vi "Gamepad NanoDrive Control.vi"() -> ()   [LabVIEW 2012]
uses:
  <vilib>/Utility/miscctls.llb/LVPointTypeDef.ctl
  <vilib>/Utility/file.llb/Read From Spreadsheet File (I64).vi
  <vilib>/Utility/inputDevices.llb/joystickAcquire.vi
  <vilib>/Utility/inputDevices.llb/closeJoystick.vi
  Madlib.dll
panel:
  out "Y axis":dbl
  out "X axis":dbl
  out "yRead":dbl=5.0 step=0.1 format="%.3f"
  out "xRead":dbl=5.0 step=0.1 format="%.3f"
  in  "left":bool
  in  "down":bool
  in  "right":bool
  in  "up":bool
  in  "closed?":bool
  in  "Slide":cluster{u32, u32}(slide)={0, 5} scale=0.0..7.0
  in  "configure":bool
  out "button selection refs":T1
  in  "yf":u16(ring)=4 items=["1 X"=1, "2 A"=2, "3 B"=3, "4 Y"=4, "5 LB"=5, "6 RB"=6, "7 LT"=7, "8 RT"=8, "9 Back"=9]
  in  "xf":u16(ring)=3 items=["1 X"=1, "2 A"=2, "3 B"=3, "4 Y"=4, "5 LB"=5, "6 RB"=6, "7 LT"=7, "8 RT"=8, "9 Back"=9]
  in  "yf xr 2":u16(ring)=5 items=["1 X"=1, "2 A"=2, "3 B"=3, "4 Y"=4, "5 LB"=5, "6 RB"=6, "7 LT"=7, "8 RT"=8, "9 Back"=9]
  in  "halt 3":u16(ring)=9 items=["1 X"=1, "2 A"=2, "3 B"=3, "4 Y"=4, "5 LB"=5, "6 RB"=6, "7 LT"=7, "8 RT"=8, "9 Back"=9]
  in  "yf xf 2":u16(ring)=6 items=["1 X"=1, "2 A"=2, "3 B"=3, "4 Y"=4, "5 LB"=5, "6 RB"=6, "7 LT"=7, "8 RT"=8, "9 Back"=9]
  in  "yr xr 2":u16(ring)=7 items=["1 X"=1, "2 A"=2, "3 B"=3, "4 Y"=4, "5 LB"=5, "6 RB"=6, "7 LT"=7, "8 RT"=8, "9 Back"=9]
  in  "yr":u16(ring)=2 items=["1 X"=1, "2 A"=2, "3 B"=3, "4 Y"=4, "5 LB"=5, "6 RB"=6, "7 LT"=7, "8 RT"=8, "9 Back"=9]
  in  "yr xf 2":u16(ring)=8 items=["1 X"=1, "2 A"=2, "3 B"=3, "4 Y"=4, "5 LB"=5, "6 RB"=6, "7 LT"=7, "8 RT"=8, "9 Back"=9]
  in  "xr":u16(ring)=1 items=["1 X"=1, "2 A"=2, "3 B"=3, "4 Y"=4, "5 LB"=5, "6 RB"=6, "7 LT"=7, "8 RT"=8, "9 Back"=9]
  in  "down-left":bool
  in  "down-right":bool
  in  "up-left":bool
  in  "up-right":bool
  in  "yStep":dbl=1.0 min=0.01905 max=4.0 format="%.3f"
  in  "xStep":dbl=1.0 min=0.01905 max=4.0 format="%.3f"
  in  "Invert":bool=TRUE
  in  "Invert":bool
  # "Single Step Controls"
  # "Position"
  # "Step distance"
  # "Current position"
  # "X axis"
  # "X axis"
  # "um"
  # "um"
  # "Y axis"
  # "Y axis"
  # "um"
  # "um"
  # "Step"
  # "Commanded position"
  # "um"
  # "um"
  # "Configuration"
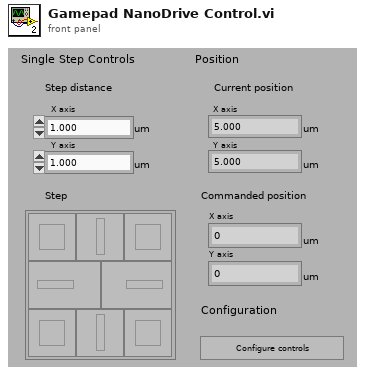
[diagram p1: front panel]
types:
  T1 = cluster{"xr":refnum<vi>, "yr":refnum<vi>, "xf":refnum<vi>, "yf":refnum<vi>, "yf xr 2":refnum<vi>, "yf xf 2":refnum<vi>, "yr xr 2":refnum<vi>, "yr xf 2":refnum<vi>, "halt 2":refnum<vi>}
  T2 = enum16{"open", "replace", "create", "open or create", "replace or create", "replace or create with confirmation"}
  T3 = typedef "LVPointTypeDef.ctl" = cluster{"Horizontal":i16, "Vertical":i16}
  T4 = cluster{"Controls":cluster{"Commands":cluster{"unused":bool}, "Values":cluster{"up":u16, "right":u16}}, "ControlRefs":cluster{"Commands":cluster{"unused":refnum<vi>}, "Values":cluster{"up":refnum<vi>, "right":refnum<vi>}}, "Variables":cluster{"Commands":cluster{"up_changed":bool, "right_changed":bool}, "Values":cluster{"unused":i32}}}
  T5 = cluster{"Controls":cluster{"Commands":cluster{"right":bool, "left":bool, "up":bool, "down":bool, "down-left":bool, "up-left":bool, "up-right":bool, "down-right":bool}, "Values":cluster{"xStep":dbl, "yStep":dbl, "xRead":dbl, "yRead":dbl}}, "ControlRefs":cluster{"Commands":cluster{"right":refnum<vi>, "left":refnum<vi>, "up":refnum<vi>, "down":refnum<vi>, "down-left":refnum<vi>, "up-left":refnum<vi>, "up-right":refnum<vi>, "down-right":refnum<vi>}, "Values":cluster{"X step":refnum<vi>, "Y step":refnum<vi>, "xRead":refnum<vi>, "yRead":refnum<vi>}}, "Variables":cluster{"Commands":cluster{"unused":bool}, "Values":cluster{"xCommand":dbl, "yCommand":dbl, "xCalibration":dbl, "yCalibration":dbl}}}
  T6 = cluster{"xr":refnum<vi>, "yr":refnum<vi>, "xf":refnum<vi>, "yf":refnum<vi>, "yf xr 2":refnum<vi>, "yf xf 2":refnum<vi>, "yr xr 2":refnum<vi>, "yr xf 2":refnum<vi>, "halt 3":refnum<vi>}
  T7 = cluster{"X axis":i32, "Y axis":i32, "Z axis":i32, "X axis rotation":i32, "Y axis rotation":i32, "Z axis rotation":i32, "U axis":i32, "V axis":i32}
  T8 = cluster{"button 1":bool, "button 2":bool, "button 3":bool, "button 4":bool, "button 5":bool, "button 6":bool, "button 7":bool, "button 8":bool, "button 9":bool, "button 10":bool, "button 11":bool, "button 12":bool, "button 13":bool, "button 14":bool, "button 15":bool, "button 16":bool, "button 17":bool, "button 18":bool, "button 19":bool, "button 20":bool, "button 21":bool, "button 22":bool, "button 23":bool, "button 24":bool, "button 25":bool, "button 26":bool, "button 27":bool, "button 28":bool, "button 29":bool, "button 30":bool, "button 31":bool, "button 32":bool}
  T9 = cluster{"left":bool, "down":bool, "right":bool, "up":bool, "up-left":bool, "up-right":bool, "down-left":bool, "down-right":bool, "halt":bool, "button 10":bool}
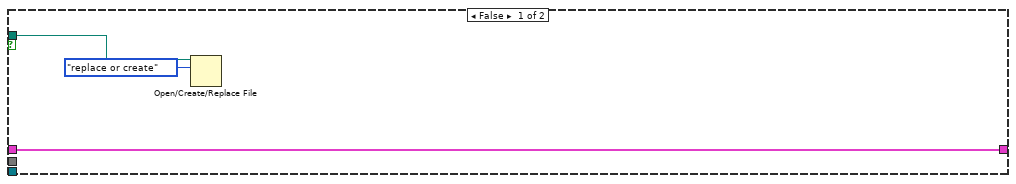
[diagram p2: hidden frame]
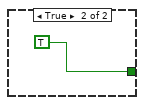
[diagram p4: hidden frame]
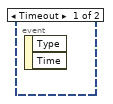
[diagram p8: hidden frame]
diagram:
  n1 = flat-sequence {
    tunnel: [w44] -> w25
    tunnel: [w43] -> w24
    tunnel: [w42] -> w23
    tunnel: [w61] -> w17
    tunnel: [w60] -> w16
    tunnel: [w59] -> w15
    tunnel: w25 -> [w61]
    tunnel: w24 -> [w56]
    tunnel: w23 -> [w59]
    tunnel: w17 -> [w64]
    tunnel: [w63] -> w27
    tunnel: w16 -> [w74]
    tunnel: [w74] -> w26
    tunnel: w15 -> [w62]
    tunnel: [w62] -> w22
    tunnel: w27 -> [w80]
    tunnel: [w80] -> w29
    tunnel: w26 -> [w86]
    tunnel: [w86] -> w28
    tunnel: w22 -> [w77]
    tunnel: [w76] -> w19
    tunnel: [w135] -> w35
    tunnel: [w136] -> w31
    tunnel: w28 -> [w136]
    tunnel: w29 -> [w135]
    tunnel: [w128] -> w20
    tunnel: w19 -> [w128]
    tunnel: [w141] -> w38
    tunnel: [w140] -> w37
    tunnel: w35 -> [w139]
    tunnel: [w139] -> w34
    tunnel: [w138] -> w32
    tunnel: w31 -> [w138]
    tunnel: [w137] -> w21
    tunnel: w20 -> [w137]
    tunnel: [w167] -> w12
    tunnel: [w168] -> w10
    tunnel: [w164] -> w8
    tunnel: w38 -> [w168]
    tunnel: w37 -> [w167]
    tunnel: w34 -> [w163]
    tunnel: [w163] -> w6
    tunnel: w32 -> [w162]
    tunnel: [w162] -> w4
    tunnel: w21 -> [w161]
    tunnel: [w161] -> w2
    tunnel: w12 -> [w190]
    tunnel: [w190] -> w11
    tunnel: w10 -> [w189]
    tunnel: [w189] -> w9
    tunnel: w8 -> [w185]
    tunnel: [w185] -> w7
    tunnel: w6 -> [w184]
    tunnel: [w184] -> w5
    tunnel: w4 -> [w183]
    tunnel: [w180] -> w3
    tunnel: w2 -> [w188]
    tunnel: [w188] -> w1
    tunnel: w11 -> [w197]
    tunnel: [w197] -> w41
    tunnel: w9 -> [w198]
    tunnel: [w198] -> w40
    tunnel: w7 -> [w196]
    tunnel: [w196] -> w39
    tunnel: [u32 0 ("current button state")] -> w36
    tunnel: [w193] -> w33
    tunnel: w5 -> [w193]
    tunnel: [w192] -> w30
    tunnel: w3 -> [w192]
    tunnel: [w191] -> w18
    tunnel: w1 -> [w191]
    tunnel: w39 -> [w205]
    tunnel: w40 -> [w207]
    tunnel: w41 -> [w206]
    tunnel: w36 -> [w204]
    tunnel: w33 -> [w203]
    tunnel: w30 -> [w202]
    tunnel: w18 -> [w201]
    tunnel: [w200] -> w14
    tunnel: [w199] -> w13
    tunnel: w14 -> [w489]
    tunnel: w13 -> [w488]
    frame #0 {
      w42 = T4 {"Controls"={"Commands"={"unused"=FALSE}, "Values"={"up"=2, "right"=0}}, "ControlRefs"={"Commands"={"unused"=refnum}, "Values"={"up"=refnum, "right"=refnum}}, "Variables"={"Commands"={"up_changed"=FALSE, "right_changed"=FALSE}, "Values"={"unused"=0}}}  # Configuration
      w43 = T5 {"Controls"={"Commands"={"right"=FALSE, "left"=FALSE, "up"=FALSE, "down"=FALSE, "down-left"=FALSE, "up-left"=FALSE, "up-right"=FALSE, "down-right"=FALSE}, "Values"={"xStep"=1.0, "yStep"=1.0, "xRead"=1.0, "yRead"=1.0}}, "ControlRefs"={"Commands"={"right"=refnum, "left"=refnum, "up"=refnum, "down"=refnum, "down-left"=refnum, "up-left"=refnum, "up-right"=refnum, "down-right"=refnum}, "Values"={"X step"=refnum, "Y step"=refnum, "xRead"=refnum, "yRead"=refnum}}, "Variables"={"Commands"={"unused"=FALSE}, "Values"={"xCommand"=0.0, "yCommand"=0.0, "xCalibration"=0.0, "yCalibration"=0.0}}}  # Motion
      w44 = T6 {"xr"=refnum, "yr"=refnum, "xf"=refnum, "yf"=refnum, "yf xr 2"=refnum, "yf xf 2"=refnum, "yr xr 2"=refnum, "yr xf 2"=refnum, "halt 3"=refnum}  # output cluster
    }
    frame #1 {
      n2 = control-ref of="right"() -> (w54:refnum<vi>)
      n3 = control-ref of="left"() -> (w53:refnum<vi>)
      n4 = control-ref of="up"() -> (w52:refnum<vi>)
      n5 = control-ref of="down"() -> (w51:refnum<vi>)
      n6 = control-ref of="down-left"() -> (w50:refnum<vi>)
      n7 = control-ref of="up-left"() -> (w49:refnum<vi>)
      n8 = control-ref of="up-right"() -> (w48:refnum<vi>)
      n9 = control-ref of="down-right"() -> (w47:refnum<vi>)
      n10 = control-ref of="xStep"() -> (w57:refnum<vi>)
      n11 = control-ref of="yStep"() -> (w58:refnum<vi>)
      n12 = control-ref of="xRead"() -> (w46:refnum<vi>)
      n13 = control-ref of="yRead"() -> (w45:refnum<vi>)
      n14 = Bundle By Name(cluster=w56, "ControlRefs.Values.X step"=w57, "ControlRefs.Values.Y step"=w58, "ControlRefs.Values.xRead"=w46, "ControlRefs.Values.yRead"=w45) -> (w55:T5)
      n15 = Bundle By Name(cluster=w55, "ControlRefs.Commands.right"=w54, "ControlRefs.Commands.left"=w53, "ControlRefs.Commands.up"=w52, "ControlRefs.Commands.down"=w51, "ControlRefs.Commands.down-left"=w50, "ControlRefs.Commands.up-left"=w49, "ControlRefs.Commands.up-right"=w48, "ControlRefs.Commands.down-right"=w47) -> (w60:T5)
    }
    frame #2 {
      n16 = control-ref of="xr"() -> (w73:refnum<vi>)
      n17 = control-ref of="yr"() -> (w72:refnum<vi>)
      n18 = control-ref of="xf"() -> (w71:refnum<vi>)
      n19 = control-ref of="yf"() -> (w70:refnum<vi>)
      n20 = control-ref of="yf xr 2"() -> (w69:refnum<vi>)
      n21 = control-ref of="yf xf 2"() -> (w68:refnum<vi>)
      n22 = control-ref of="yr xr 2"() -> (w67:refnum<vi>)
      n23 = control-ref of="yr xf 2"() -> (w66:refnum<vi>)
      n24 = control-ref of="halt 3"() -> (w65:refnum<vi>)
      n25 = Bundle(cluster=w64, "xr"=w73, "yr"=w72, "xf"=w71, "yf"=w70, "yf xr 2"=w69, "yf xf 2"=w68, "yr xr 2"=w67, "yr xf 2"=w66, "halt 3"=w65) -> (w63:T6)
    }
    frame #3 {
      n26 = control-ref of="This Application"() -> (w85:refnum<vi>)
      n27 = property class="App"(reference=w85) -> ("App.Dir"=w79:path)  [unwired: 1 in, 2 out]
      n28 = control-ref of="Slide"() -> (w82:refnum<vi>)
      n29 = Build Path(base path=w79, name or relative path="config.txt") -> (appended path=w83:path)
      n30 = Cluster To Array(cluster=w80) -> (array=w81:refnum<vi>[])
      n31 = call <vilib>:"Check if File or Folder Exists.vi"("path"=w83) -> ("file or folder exists?"=w75:bool, "dup path"=w78:path)  [unwired: 1 in, 8 out]
      n32 = case shown="True" w75 {
        tunnel: w82 -> [_ w103]
        tunnel: w81 -> [_ w102]
        tunnel: w78 -> [w89 w101]
        tunnel: w77 -> [w87 w91]
        tunnel: [w87 w90] -> w76
        frame False {
          n33 = Open/Create/Replace File(file path (use dialog)=w89, operation (0:open)=T2."replace or create") -> ()  [unwired: 1 in, 6 out]
        }
        frame True {
          n34 = Read from Text File(file (use dialog)=w101) -> (text=w100:string)  [unwired: 1 in, 5 out]
          n35 = String To Path(string=w100) -> (path=w99:path)
          n36 = call <vilib>:"Check if File or Folder Exists.vi"("path"=w99) -> ("file or folder exists?"=w97:bool, "dup path"=w93:path)  [unwired: 1 in, 8 out]
          n37 = Not A Number/Path/Refnum?(number/path/refnum=w93) -> (NaN/Path/Refnum?=w96:bool)
          n38 = Empty String/Path?(string/path=w93) -> (empty?=w94:bool)
          n39 = Not(x=w96) -> (.not. x?=w95:bool)
          n40 = Not(x=w94) -> (.not. x?=w92:bool)
          n41 = Compound Arithmetic op=AND(w95, w97, w92) -> (w98:bool)
          n42 = case shown="True" w98 {
            tunnel: w102 -> [_ w122]
            tunnel: w103 -> [_ w123]
            tunnel: w93 -> [_ w121]
            tunnel: w91 -> [w104 w120]
            tunnel: [w104 w119] -> w90
            frame False {
            }
            frame True {
              n43 = call-poly <vilib>:"Read From Spreadsheet File.vi"("transpose (no:F)"=TRUE ("transpose? (no:F)"), "file path (dialog if empty)"=w121) -> ("first row"=w124:i64[])  [unwired: 2 in, 7 out]
              n44 = Array Size(array=w122) -> (size(s)=w118:i32)
              n45 = Split 1D Array(array=w124, index=w118) -> (first subarray=w115:i64[], second subarray=w117:i64[])
              n46 = Index Array(array=w117) -> (element #1=w107:i64, element #2=w108:i64, element #3=w114:i64, element #4=w111:i64, element #5=w106:i64, element #6=w105:i64)  [unwired: 6 in]
              n47 = Bundle(w108, w107) -> (w116:cluster{i64, i64})  [unwired: 1 out]
              n48 = property class="Slide (strict)"(reference=w123, "Value"=w116) -> ()  [unwired: 1 in, 2 out]
              n49 = Bundle By Name(cluster=w120, "Controls.Values.up"=w106, "Controls.Values.right"=w105) -> (w119:T4)
              n50 = control-ref of="Invert"() -> (w110:refnum<vi>)
              n51 = control-ref of="Invert"() -> (w109:refnum<vi>)
              n52 = Greater Than 0?(x=w114) -> (x > 0?=w113:bool)
              n53 = Greater Than 0?(x=w111) -> (x > 0?=w112:bool)
              n54 = property class="Bool (strict)"(reference=w110, "Value"=w113) -> ()  [unwired: 1 in, 2 out]
              n55 = property class="Bool (strict)"(reference=w109, "Value"=w112) -> ()  [unwired: 1 in, 2 out]
              n56 = for {
                tunnel: w122 -> [w127] mode=indexing
                tunnel: w115 -> [w126] mode=indexing
                n57 = property class="Ring (strict)"(reference=w127, "Value"=w126) -> ()  [unwired: 1 in, 2 out]
              }
            }
          }
        }
      }
    }
    frame #4 {
      w131 = TRUE ("Front Panel Window:Closeable")
      w132 = FALSE ("Front Panel Window:Title Bar Visible")
      n58 = control-ref of="Pane"() -> (w129:refnum<vi>)
      n59 = control-ref of="This VI"() -> (w134:refnum<vi>)
      n60 = property class="VI"(reference=w134, "Front Panel.Title"="Gamepad NanoDrive Control" ("Front Panel Window:Title"), "Front Panel.TitleBarVis"=w131, "TB.Visible"=w132, "Front Panel.ShowMenuBar"=w132, "Front Panel.Closeable"=w131) -> ()  [unwired: 1 in, 2 out]
      n61 = property class="Pane"(reference=w129, "Origin"=T3 {"Horizontal"=0, "Vertical"=0}) -> ()  [unwired: 1 in, 2 out]
    }
    frame #5 {
      n62 = while {
        tunnel: [w147] -> w140
        tunnel: [w142] -> w141
        stop <- w146 stop-if-true
        n63 = flat-sequence {
          tunnel: [w150] -> w149
          tunnel: [w151] -> w148
          tunnel: [w150] -> w145
          tunnel: w149 -> [w155]
          tunnel: [w154] -> w147
          tunnel: w148 -> [w154]
          tunnel: [w153] -> w142
          tunnel: w145 -> [w153]
          tunnel: [w152] -> w144
          frame #0 {
            n64 = call "init joystick.vi"() -> ("device ID"=w151:refnum<k1>, "Joystick found"=w150:bool)  [unwired: 2 out]
          }
          frame #1 {
            n65 = case shown="False" w155 {
              tunnel: [w156 TRUE ("T button?")] -> w152
              frame False {
                n66 = Two Button Dialog(message="Press start (button 10)\n on your Gamepad \n(while pressing 'Ok')\nfor it to be initialized. ", 1:"Cancel Program" ("F button name (\"Cancel\")"), 2:"Ok" ("T button name (\"OK\")")) -> (T button?=w156:bool)
              }
              frame True {
              }
            }
          }
        }
        n67 = Not(x=w144) -> (.not. x?=w143:bool)
        n68 = Or(x=w143, y=w142) -> (x .or. y?=w146:bool)
      }
    }
    frame #6 {
      n69 = dll-call lib="C:/Users/Labview/Desktop/SRR/Madlib_x64/Labview Examples/Madlib.dll" fn="MCL_InitHandleOrGetExisting"() -> ("return type"=w165:i32)  [unwired: 3 in, 2 out]
      n70 = Less Or Equal To 0?(x=w165) -> (x <= 0?=w166:bool)
      n71 = case shown="True" w166 {
        tunnel: w165 -> [w169 w171]
        tunnel: [w169 w170] -> w164
        frame False {
        }
        frame True {
          n72 = while {
            tunnel: w171 -> [w176]
            tunnel: [w174] -> w170
            stop <- w173 continue-if-true
            n73 = Two Button Dialog(message="Failed to load NanoDrive!\nReInit?") -> (T button?=w172:bool)  [unwired: 2 out]
            n74 = case shown="True" w172 {
              tunnel: w176 -> [w178 _]
              tunnel: [w178 w179] -> w174
              frame False {
              }
              frame True {
                n75 = dll-call lib="C:/Users/Labview/Desktop/SRR/Madlib_x64/Labview Examples/Madlib.dll" fn="MCL_InitHandleOrGetExisting"() -> ("return type"=w179:i32)  [unwired: 3 in, 2 out]
              }
            }
            n76 = Less Or Equal To 0?(x=w174) -> (x <= 0?=w175:bool)
            n77 = And(x=w172, y=w175) -> (x .and. y?=w173:bool)
          }
        }
      }
    }
    frame #7 {
      n78 = dll-call lib="C:/Users/Labview/Desktop/SRR/Madlib_x64/Labview Examples/Madlib.dll" fn="MCL_GetCalibration" ("MADLib.dll:MCL_InitHandleOrGetExisting")("axis"=1, "handle"=w185) -> ("calibration"=w182:dbl)  [unwired: 3 in, 4 out]
      n79 = dll-call lib="C:/Users/Labview/Desktop/SRR/Madlib_x64/Labview Examples/Madlib.dll" fn="MCL_GetCalibration" ("MADLib.dll:MCL_InitHandleOrGetExisting")("axis"=2, "handle"=w185) -> ("calibration"=w181:dbl)  [unwired: 3 in, 4 out]
      n80 = Bundle By Name(cluster=w183, "Variables.Values.xCalibration"=w182, "Variables.Values.yCalibration"=w181) -> (w180:T5)
    }
    frame #8 {
      n81 = local write "closed?"(FALSE ("closed?")) -> ()
    }
    frame #9 {
      n82 = case shown="True" w207 {
        tunnel: w206 -> [_ w216]
        tunnel: w205 -> [_ w215]
        tunnel: w204 -> [_ w213]
        tunnel: w203 -> [_ w212]
        tunnel: w202 -> [_ w208]
        tunnel: w201 -> [_ w211]
        tunnel: [_ w210] -> w200
        tunnel: [_ w209] -> w199
        frame False {
        }
        frame True {
          n83 = while {
            tunnel: w216 -> [w314]
            tunnel: [w313] -> w209
            tunnel: [w312] -> w210
            tunnel: w215 -> [w311]
            shift-right: [w310] -> _
            shift-left: w213 -> [w309]
            tunnel: w212 -> [w301]
            shift-right: [w280] -> _
            shift-left: w211 -> [w285]
            shift-right: [w267] -> _
            shift-left: w208 -> [w266]
            stop <- w308 stop-if-true
            n84 = Wait Until Next ms Multiple(millisecond multiple=u32 10) -> ()  [unwired: 1 out]
            n85 = flat-sequence {
              tunnel: [w329] -> w279
              tunnel: [w328] -> w278
              tunnel: [w327] -> w277
              tunnel: [w326] -> w276
              tunnel: [w325] -> w275
              tunnel: [w324] -> w274
              tunnel: w309 -> [w329]
              tunnel: w311 -> [w328]
              tunnel: w314 -> [w327]
              tunnel: w301 -> [w326]
              tunnel: w285 -> [w324]
              tunnel: w266 -> [w315]
              tunnel: [w338] -> w273
              tunnel: [w337] -> w272
              tunnel: [w336] -> w271
              tunnel: [w333] -> w270
              tunnel: [w335] -> w269
              tunnel: [w334] -> w268
              tunnel: w274 -> [w334]
              tunnel: w275 -> [w332]
              tunnel: w276 -> [w333]
              tunnel: w277 -> [w336]
              tunnel: w278 -> [w337]
              tunnel: w279 -> [w338]
              tunnel: [w348] -> w307
              tunnel: [w347] -> w305
              tunnel: [w346] -> w303
              tunnel: [w345] -> w299
              tunnel: w273 -> [w348]
              tunnel: w272 -> [w347]
              tunnel: w271 -> [w346]
              tunnel: w270 -> [w345]
              tunnel: [w341] -> w292
              tunnel: w269 -> [w341]
              tunnel: w268 -> [w344]
              tunnel: [w344] -> w283
              tunnel: w307 -> [w356]
              tunnel: [w356] -> w306
              tunnel: w305 -> [w355]
              tunnel: [w355] -> w304
              tunnel: w303 -> [w353]
              tunnel: [w353] -> w302
              tunnel: [w352] -> w300
              tunnel: w299 -> [w352]
              tunnel: [w351] -> w293
              tunnel: w292 -> [w351]
              tunnel: [w349] -> w284
              tunnel: w283 -> [w350]
              tunnel: [w375] -> w290
              tunnel: [w368] -> w289
              tunnel: [w374] -> w288
              tunnel: [w373] -> w287
              tunnel: [w370] -> w286
              tunnel: [w372] -> w282
              tunnel: w284 -> [w372]
              tunnel: w293 -> [w371]
              tunnel: w300 -> [w373]
              tunnel: w302 -> [w375]
              tunnel: w304 -> [w368]
              tunnel: w306 -> [w374]
              tunnel: [w383] -> w298
              tunnel: [w382] -> w297
              tunnel: [w381] -> w296
              tunnel: [w377] -> w295
              tunnel: [w380] -> w294
              tunnel: [w379] -> w291
              tunnel: [w378] -> w281
              tunnel: [w376] -> w255
              tunnel: w290 -> [w383]
              tunnel: w289 -> [w382]
              tunnel: w288 -> [w381]
              tunnel: w287 -> [w376]
              tunnel: w286 -> [w379]
              tunnel: w282 -> [w378]
              tunnel: [w416] -> w261
              tunnel: [w417] -> w262
              tunnel: [w415] -> w263
              tunnel: [w414] -> w264
              tunnel: [w413] -> w265
              tunnel: [w412] -> w260
              tunnel: [w411] -> w259
              tunnel: [w410] -> w258
              tunnel: w281 -> [w413]
              tunnel: w291 -> [w414]
              tunnel: w294 -> [w385]
              tunnel: w295 -> [w412]
              tunnel: w296 -> [w415]
              tunnel: w297 -> [w417]
              tunnel: w298 -> [w416]
              tunnel: [w384] -> w256
              tunnel: w255 -> [w384]
              tunnel: [w427] -> w244
              tunnel: [w428] -> w246
              tunnel: [w430] -> w248
              tunnel: [w424] -> w250
              tunnel: [w429] -> w252
              tunnel: [w426] -> w254
              tunnel: [w425] -> w242
              tunnel: [w423] -> w236
              tunnel: [w422] -> w235
              tunnel: w256 -> [w425]
              tunnel: w258 -> [w421]
              tunnel: w259 -> [w420]
              tunnel: w260 -> [w426]
              tunnel: w261 -> [w427]
              tunnel: w262 -> [w428]
              tunnel: w263 -> [w430]
              tunnel: w264 -> [w424]
              tunnel: w265 -> [w429]
              tunnel: w254 -> [w435]
              tunnel: [w433] -> w253
              tunnel: w252 -> [w440]
              tunnel: [w440] -> w251
              tunnel: w250 -> [w439]
              tunnel: [w439] -> w249
              tunnel: w248 -> [w434]
              tunnel: [w434] -> w247
              tunnel: w246 -> [w438]
              tunnel: [w438] -> w245
              tunnel: w244 -> [w437]
              tunnel: [w437] -> w243
              tunnel: w242 -> [w436]
              tunnel: w236 -> [w431]
              tunnel: w235 -> [w432]
              tunnel: [w432] -> w234
              tunnel: [w431] -> w233
              tunnel: [w452] -> w224
              tunnel: [w445] -> w226
              tunnel: [w451] -> w228
              tunnel: [w450] -> w230
              tunnel: [w449] -> w232
              tunnel: w253 -> [w446]
              tunnel: w251 -> [w449]
              tunnel: w249 -> [w450]
              tunnel: w247 -> [w451]
              tunnel: w245 -> [w445]
              tunnel: w243 -> [w452]
              tunnel: [w444] -> w222
              tunnel: w234 -> [w444]
              tunnel: [w443] -> w221
              tunnel: w233 -> [w443]
              tunnel: [w442] -> w220
              tunnel: [w441] -> w219
              tunnel: w232 -> [w472]
              tunnel: [w472] -> w231
              tunnel: w230 -> [w458]
              tunnel: [w457] -> w229
              tunnel: w228 -> [w471]
              tunnel: [w471] -> w227
              tunnel: w226 -> [w470]
              tunnel: [w470] -> w225
              tunnel: w224 -> [w469]
              tunnel: [w469] -> w223
              tunnel: w222 -> [w456]
              tunnel: w221 -> [w455]
              tunnel: w220 -> [w454]
              tunnel: w219 -> [w453]
              tunnel: w231 -> [w481]
              tunnel: [w481] -> w241
              tunnel: w229 -> [w475]
              tunnel: [w475] -> w240
              tunnel: w227 -> [w480]
              tunnel: [w480] -> w239
              tunnel: w225 -> [w476]
              tunnel: [w476] -> w238
              tunnel: w223 -> [w479]
              tunnel: [w479] -> w237
              tunnel: [w485] -> w310
              tunnel: [w486] -> w312
              tunnel: [w487] -> w313
              tunnel: ["closed?"] -> w308
              tunnel: [w483] -> w280
              tunnel: w241 -> [w483]
              tunnel: w240 -> [w482]
              tunnel: w239 -> [w485]
              tunnel: w238 -> [w486]
              tunnel: w237 -> [w487]
              tunnel: [w482] -> w267
              frame #0 {
                # "Update control values"
                n86 = Bundle By Name(cluster=w315, "Controls.Commands.right"="right", "Controls.Commands.left"="left", "Controls.Commands.up"="up", "Controls.Commands.down"="down", "Controls.Commands.down-left"="down-left", "Controls.Commands.up-left"="up-left", "Controls.Commands.up-right"="up-right", "Controls.Commands.down-right"="down-right") -> (w325:T5)
              }
              frame #1 {
                # "Update control values"
                n87 = Bundle By Name(cluster=w332, "Controls.Values.xStep"="xStep", "Controls.Values.yStep"="yStep") -> (w335:T5)
              }
              frame #2 {
                # "Display device info"
                n88 = Unbundle By Name(w341) -> ("Variables.Values.xCommand"=→"X axis":dbl, "Variables.Values.yCommand"=→"Y axis":dbl)
                n89 = Unbundle By Name(w341) -> ("Controls.Values.xRead"=→"xRead":dbl, "Controls.Values.yRead"=→"yRead":dbl)
              }
              frame #3 {
                # "Configure the Gamepad control stick and buttons."
                n90 = case shown="True" "configure" {
                  tunnel: w353 -> [_ w361]
                  tunnel: w352 -> [_ w360]
                  tunnel: w350 -> [w357 w359]
                  tunnel: [w357 w358] -> w349
                  frame False {
                  }
                  frame True {
                    n91 = control-ref of="Invert"() -> (w363:refnum<vi>)
                    n92 = control-ref of="Invert"() -> (w362:refnum<vi>)
                    n93 = control-ref of="Slide"() -> (w364:refnum<vi>)
                    n94 = call "Configure Gamepad.vi"("Cluster"=w360, "Configuration"=w359, "Slide 2"=w364, "invert y"=w362, "invert x"=w363, "device ID"=w361) -> ("Configuration"=w358:T4)  [unwired: 5 out]
                  }
                }
              }
              frame #4 {
                # "Read the ADCs"
                n95 = dll-call lib="C:/Users/Labview/Desktop/SRR/Madlib_x64/Labview Examples/Madlib.dll" fn="MCL_SingleReadN"("axis"=1, "handle"=w368) -> ("position"=w366:dbl)  [unwired: 4 in, 3 out]
                n96 = dll-call lib="C:/Users/Labview/Desktop/SRR/Madlib_x64/Labview Examples/Madlib.dll" fn="MCL_SingleReadN"("axis"=2, "handle"=w368) -> ("position"=w365:dbl)  [unwired: 4 in, 3 out]
                n97 = Bundle By Name(cluster=w371, "Controls.Values.xRead"=w366, "Controls.Values.yRead"=w365) -> (w370:T5)
              }
              frame #5 {
                # "Get the Gamepad info"
                n98 = call-poly <vilib>:"Acquire Input Data.vi"("device ID"=w383) -> ("axis info"=w380:T7, "button info"=w377:T8)  [unwired: 1 in, 16 out]
              }
              frame #6 {
                w407 = 0.05 ("return type")
                w408 = 0.05 ("return type")
                # "Get a number from -1 to 1 representing the control-stick position"
                n99 = Cluster To Array(cluster=w385) -> (array=w390:i32[])
                n100 = Unbundle("Slide") -> (w388:u32, w387:u32)
                n101 = Index Array(array=w390, index #1=w388, index #2=w387) -> (element #1=w391:i32, element #2=w386:i32)
                n102 = Negate(x=w386) -> (-x=w393:i32)
                n103 = Negate(x=w391) -> (-x=w403:i32)
                n104 = Select(t=w393, s="Invert", f=w386) -> (s? t:f=w405:i32)
                n105 = Select(t=w403, s="Invert", f=w391) -> (s? t:f=w404:i32)
                n106 = Divide(x=w404, y=32768) -> (x/y=w395:dbl)
                n107 = Negate(x=w408) -> (-x=w409:dbl)
                n108 = Divide(x=w405, y=32768) -> (x/y=w394:dbl)
                n109 = Negate(x=w407) -> (-x=w406:dbl)
                n110 = In Range and Coerce(upper limit=w408, x=w394, lower limit=w409) -> (In Range?=w399:bool)  [unwired: 1 out]
                n111 = In Range and Coerce(upper limit=w407, x=w395, lower limit=w406) -> (In Range?=w397:bool)  [unwired: 1 out]
                n112 = Select(t=0.0, s=w397, f=w395) -> (s? t:f=w410:dbl)
                n113 = Select(t=0.0, s=w399, f=w394) -> (s? t:f=w411:dbl)
              }
              frame #7 {
                # "Change the -1 to 1 control-stick value to something much smaller"
                n114 = Divide(x=w421, y=100.0) -> (x/y=w423:dbl)
                n115 = Divide(x=w420, y=100.0) -> (x/y=w422:dbl)
              }
              frame #8 {
                # "Have any Gamepad buttons been pressed?"
                n116 = call "user maped buttons.vi"("previous button state"=w434, "gp button info"=w435, "map references"=w436) -> ("mapped gp buttons"=w433:T9)  [unwired: 2 out]
              }
              frame #9 {
                n117 = Unbundle By Name(w450) -> ("Controls.Values.xStep"=w447:dbl, "Controls.Values.yStep"=w448:dbl)
                n118 = call "button commands.vi"("Configuration"=w449, "Motion"=w450, "Y Steps"=w448, "mapped gp buttons"=w446, "X Steps"=w447) -> ("Y distance"=w441:dbl, "X distance"=w442:dbl)  [unwired: 5 out]
              }
              frame #10 {
                n119 = Unbundle By Name(w458) -> ("Variables.Values.xCalibration"=w464:dbl, "Variables.Values.xCommand"=w468:dbl, "Variables.Values.yCommand"=w467:dbl, "Variables.Values.yCalibration"=w460:dbl)
                n120 = Compound Arithmetic op=ADD(w468, w455, w454) -> (w466:dbl)
                n121 = Compound Arithmetic op=ADD(w467, w456, w453) -> (w462:dbl)
                n122 = In Range and Coerce(upper limit=w464, x=w466, lower limit=0.0) -> (coerced(x)=w465:dbl)  [unwired: 1 out]
                n123 = In Range and Coerce(upper limit=w460, x=w462, lower limit=0.0) -> (coerced(x)=w459:dbl)  [unwired: 1 out]
                n124 = Bundle By Name(cluster=w458, "Variables.Values.xCommand"=w465, "Variables.Values.yCommand"=w459) -> (w457:T5)
              }
              frame #11 {
                n125 = Unbundle By Name(w475) -> ("Variables.Values.xCommand"=w474:dbl, "Variables.Values.yCommand"=w473:dbl)
                n126 = dll-call lib="C:/Users/Labview/Desktop/SRR/Madlib_x64/Labview Examples/Madlib.dll" fn="MCL_SingleWriteN"("command"=w473, "axis"=2, "handle"=w476) -> ()  [unwired: 4 in, 5 out]
                n127 = dll-call lib="C:/Users/Labview/Desktop/SRR/Madlib_x64/Labview Examples/Madlib.dll" fn="MCL_SingleWriteN"("command"=w474, "axis"=1, "handle"=w476) -> ()  [unwired: 4 in, 5 out]
              }
              frame #12 {
              }
            }
          }
          n128 = event shown="[1] Panel Close?" {
            selector: _ -> [_ _]
            dyn-events: _ -> [_ _]
            timeout: -1 -> [_ _]
            event Timeout {
              n129 = event-data() -> ()  [unwired: 3 out]
            }
            event Panel Close? {
              n130 = event-data() -> ()  [unwired: 4 out]
              n131 = local write "closed?"(TRUE ("closed?")) -> ()
              n132 = event-data("Discard?"=TRUE) -> ()  [unwired: 1 in, 1 out]
            }
          }
        }
      }
    }
    frame #10 {
      n133 = call-poly <vilib>:"Close Input Device.vi"("device ID"=w488) -> ()  [unwired: 1 in, 9 out]
      n134 = dll-call lib="C:/Users/Labview/Desktop/SRR/Madlib_x64/Labview Examples/Madlib.dll" fn="MCL_ReleaseHandle"("handle"=w489) -> ()  [unwired: 4 in, 3 out]
    }
  }
